vi "SVFA Get Waterfall Value (Scalar X).vi"(0 "waterfall data":T1, 2 "x value (1000)":dbl=1000.0, 3 "coercion (nearest)":T8(ring), 4 "spectrum info":T2 {"x-axis units" items=["Time (s)"=0, "Frequency-CB (Hz)"=1, "Frequency-CPB (Hz)"=1248, "Frequency-Arbitrary (Hz)"=2357, "Quefrency (s)"=2, "Revolutions (rev)"=3, "Order"=4, "Speed (RPM)"=11, "Speed (rad/s)"=21, "Index"=65535]; "weighting filter" items=["Linear", "A-weighting", "B-weighting", "C-weighting", "ITU-R 468-4", "Dolby", "CCITT", "C-message", "Wb", "Wc", "Wd", "We", "Wf", "Wh", "Wj", "Wk", "Wm", "AES17 20 kHz lowpass", "AES17 40 kHz lowpass", "AES17 20 kHz highpass", "AES17 40 kHz highpass"]; "dB reference [EU]" format="%.2f"; "engineering units" items=["custom..."=0, "V"=1, "A"=21, "C"=30, "pC"=31, "s"=32, "-"=29, "Pa"=2, "N"=20, "g"=3, "m/s^2"=4, "m/s"=5, "m"=6, "mm/s"=12, "mm"=13, "micron/s"=14, "micron"=15, "in/s^2"=7, "in/s"=8, "in"=9, "mil/s"=10, "mil"=11, "rad/s^2"=16, "rad/s"=17, "rad"=18, "deg/s^2"=26, "deg/s"=27, "deg"=28, "RPM"=22, "cycle/s^2"=23, "Hz"=24, "cycle"=25, "strain"=19]; "spectral info"."window" items=["None "=0, "Hanning"=1, "Hamming"=2, "Blackman-Harris"=3, "Exact Blackman"=4, "Blackman"=5, "Flat Top"=6, "4 Term B-Harris "=7, "7 Term B-Harris"=8, "Low Sidelobe"=9, "Force - Exponential"=10, "Gaussian"=62]}, 5 "error in":errorcluster) -> (14 "waterfall values":cluster{"X":dbl, "Y":dbl, "Z":dbl}[](array[cluster]), 19 "error out":errorcluster)   [LabVIEW 2017]
doc: "Extracts the value of the spectrum at the specified frequency. Use the frequency coercion control to specify how the frequency should be coerced if it does not exactly coincide with a frequency line. This VI operates on any real-valued spectrum. Wire data to the <B>spectrum</B> input to determine the polymorphic instance to use or manually select the instance."
uses:
  <vilib>/addons/_NISVFA/_Shared subVIs/Controls/svc_Spectrum Info.ctl
  <vilib>/addons/_NISVFA/_Shared subVIs/Controls/svc_X-Axis Units.ctl
  <vilib>/addons/_NISVFA/_Shared subVIs/Controls/svc_Spectrum Type.ctl
  <vilib>/addons/_NISVFA/_Shared subVIs/Controls/svc_Engineering Units Text Ring.ctl
  <vilib>/addons/_NISVFA/_Shared subVIs/Controls/svc_Weighting Filter Text Ring.ctl
  <vilib>/addons/_NISVFA/_Shared subVIs/Controls/svc_Complimentary Spectrum Units.ctl
  <vilib>/addons/_NISVFA/_Spectrum Processing/SVFA Get Spectrum Value (1 Ch).vi
  <vilib>/addons/_NISVFA/_Shared subVIs/Common/svc_Spectrum Units.vi
  <vilib>/addons/_NISVFA/_Shared subVIs/Common/svc_Convert Frequency to Frequency String.vi
  <vilib>/addons/_NISVFA/_Shared subVIs/Common/svc_Get Weighting Enum and Labels.vi
  <vilib>/addons/_NISVFA/_Shared subVIs/Common/svc_Unit Label Lexical Class.vi
  <vilib>/addons/_NISVFA/_Shared subVIs/Common/svc_Engineering Units to Unit Label.vi
  <vilib>/addons/_NISVFA/_Shared subVIs/Common/svc_Format Value (DBL).vi
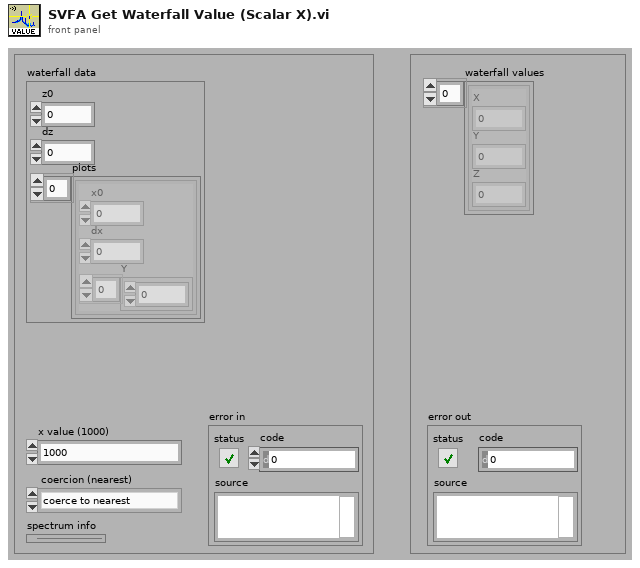
[diagram p1: front panel]
types:
  T1 = cluster{"z0":dbl, "dz":dbl, "plots":cluster{"x0":dbl, "dx":dbl, "Y":dbl[]}[]}
  T2 = typedef "svc_Spectrum Info.ctl" = cluster{"channel name":string, "description":string, "x-axis units":T3, "spectral info":cluster{"spectrum type":T4, "linear/dB":enum16{"linear", "dB"}, "window":u16, "window size":i32, "FFT size":i32}, "engineering units":T5, "custom label":string, "dB reference [EU]":dbl, "peak units":enum16{"rms", "peak", "peak-peak"}, "weighting filter":T6, "spectral density?":bool, "unit label":string, "spectrum skewed?":bool, "complimentary spectrum units":T7}
  T3 = typedef "svc_X-Axis Units.ctl" = u16
  T4 = typedef "svc_Spectrum Type.ctl" = enum16{"FFT Spectrum [complex]", "Amplitude [Magnitude]", "Power [Magnitude^2]", "Cross Spectrum [complex]", "Frequency Response [Complex]"}
  T5 = typedef "svc_Engineering Units Text Ring.ctl" = u16
  T6 = typedef "svc_Weighting Filter Text Ring.ctl" = u16
  T7 = typedef "svc_Complimentary Spectrum Units.ctl" = enum16{"none", "radians", "degrees", "cycles", "imaginary"}
  T8 = enum16{"coerce to nearest", "coerce to next highest", "coerce to next lowest", "interpolate"}
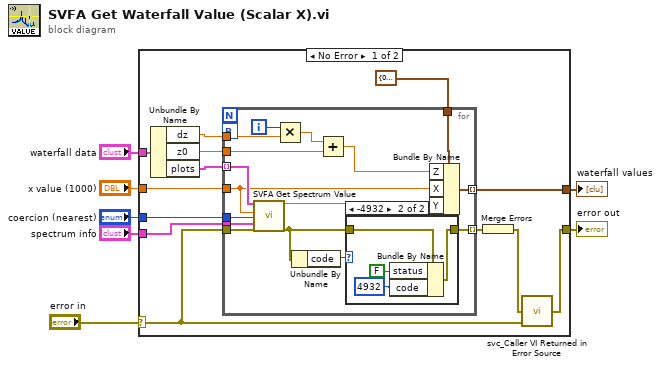
[diagram p0: block diagram]
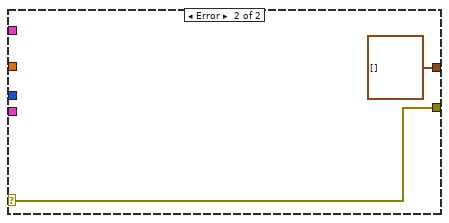
[diagram p3: hidden frame]
diagram:
  n1 = case shown="No Error" "error in" {
    selector: "error in" -> [w8 w43]
    tunnel: [w9 w43] -> w7
    tunnel: [w19 cluster{"X":dbl, "Y":dbl, "Z":dbl}[] []] -> w6
    tunnel: "coercion (nearest)" -> [w18 _]
    tunnel: "x value (1000)" -> [w17 _]
    tunnel: "spectrum info" -> [w16 _]
    tunnel: "waterfall data" -> [w15 _]
    frame No Error {
      n2 = Unbundle By Name(w15) -> ("dz"=w14:dbl, "z0"=w13:dbl, "plots"=w12:cluster{"x0":dbl, "dx":dbl, "Y":dbl[]}[])
      n3 = for {
        tunnel: w12 -> [w33] mode=indexing
        tunnel: w16 -> [w36]
        tunnel: [w34] -> w19 mode=indexing
        tunnel: cluster{"X":dbl, "Y":dbl, "Z":dbl} {"X"=0.0, "Y"=0.0, "Z"=0.0} -> [w32]
        tunnel: w17 -> [w31]
        tunnel: w18 -> [w30]
        tunnel: [w24] -> w20 mode=indexing
        tunnel: w13 -> [w26]
        tunnel: w14 -> [w25]
        workers-P: _ -> [_]
        tunnel: w8 -> [w21]
        i -> [w28]
        n4 = call-poly <vilib>:"SVFA Get Spectrum Value.vi"("spectrum"=w33, "x value (1000)"=w31, "coercion (nearest)"=w30, "spectrum info"=w36, "error in (no error)"=w21) -> ("spectrum value"=w35:dbl, "error out"=w23:errorcluster)  [unwired: 10 in, 3 out]
        n5 = Multiply(x=w28, y=w25) -> (x*y=w29:dbl)
        n6 = Unbundle By Name(w23) -> ("code"=w22:i32)
        n7 = Add(x=w29, y=w26) -> (x+y=w27:dbl)
        n8 = case shown="-4932" w22 {
          tunnel: [w37 w39] -> w24
          tunnel: w23 -> [w37 w38]
          frame Default {
          }
          frame -4932 {
            n9 = Bundle By Name(cluster=w38, "status"=FALSE, "code"=4932) -> (w39:errorcluster)
          }
        }
        n10 = Bundle By Name(cluster=w32, "Z"=w27, "X"=w31, "Y"=w35) -> (w34:cluster{"X":dbl, "Y":dbl, "Z":dbl})
      }
      n11 = Merge Errors(w20) -> (w10:errorcluster)
      n12 = call <vilib>:"svc_Caller VI Returned in Error Source.vi"("warning input to caller"=w8, "error in (no error)"=w10) -> ("error out"=w9:errorcluster)  [unwired: 3 in]
    }
    frame Error {
    }
  }
  "error out" <- w7
  "waterfall values" <- w6
